vi "Path_Menu Config Template.vi"() -> (3 "Menu Config Template path":path)   [LabVIEW 2019, in "AutoMenuCreator.lvlib"]
uses:
  AutoMenuCreator.lvlib
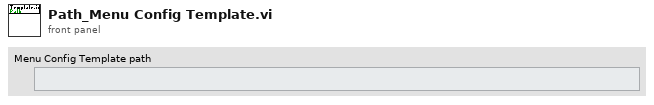
[diagram p1: front panel]
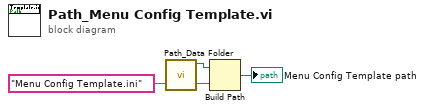
[diagram p0: block diagram]
diagram:
  n1 = call "Path_Data Folder.vi"() -> ("Data Folder Path"=w1:path)  [unwired: 11 in]
  n2 = Build Path(base path=w1, name or relative path="Menu Config Template.ini") -> (appended path=→"Menu Config Template path":path)
